vi "Init Tx Packet Size.vi"(8 "error in (no error)":errorcluster, 11 "Tx Loop Data":T1) -> (0 "error out":errorcluster, 3 "Tx Loop Data out":T1)   [LabVIEW 2016, in "UDP-Custom-Device Engine.lvlib"]
uses:
  UDP-Custom-Device Engine.lvlib
  Tx Loop Data.ctl
  <vilib>/NI Veristand/VeriStand Data/Byte Buffer/Byte Buffer.lvclass
  <vilib>/NI/NIVS Inline Async API/_Data Access Engine/Data Access Engine/Types/Read.DVR.ctl
  <vilib>/NI/NIVS Inline Async API/_Data Access Engine/Access Type Classes/Read/Read.lvclass
  <vilib>/NI Veristand/VeriStand Data/Typedefs/Typedefs.Data Types.ctl
  Data Conversion Config.ctl
  <vilib>/NI Veristand/VeriStand Data/Byte Buffer/Byte Buffer.Mapping.ctl
  Shared/Header Details.ctl
  <vilib>/NI/NIVS Inline Async API/_Data Access Engine/Data Access Engine/Data Access Engine.lvclass
  <vilib>/NI Veristand/VeriStand Data/VeriStand Data.lvlib
  Shared/UDP-Custom-Device Shared.lvlib
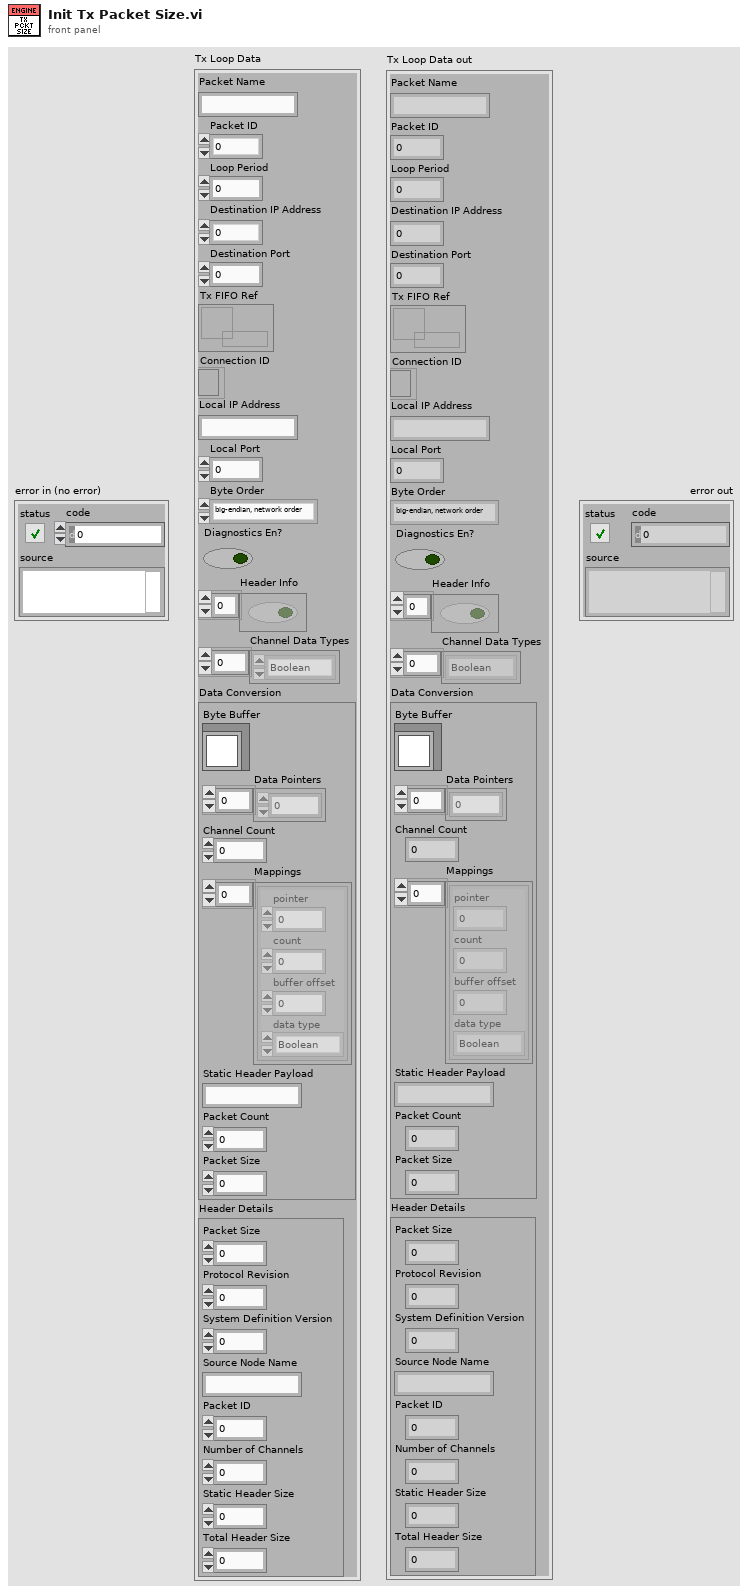
[diagram p1: front panel]
types:
  T1 = typedef "UDP-Custom-Device Engine.lvlib/Tx Loop Data.ctl" = cluster{"Packet Name":string, "Packet ID":i32, "Loop Period":u32, "Destination IP Address":u32, "Destination Port":u16, "Tx FIFO Ref":T2, "Connection ID":refnum<k16>, "Local IP Address":string, "Local Port":i32, "Byte Order":enum16{"big-endian, network order", "native, host order", "little-endian"}, "Diagnostics En?":bool, "Header Info":bool[], "Channel Data Types":T3[], "Data Conversion":T4, "Header Details":T6}
  T2 = typedef "Data Access Engine.lvlib/Data Access Engine.lvclass/Read.DVR.ctl" = refnum<data-value>
  T3 = typedef "VeriStand Data.lvlib/Typedefs.Data Types.ctl" = enum16{"Boolean", "Single", "Double", "I8", "I16", "I32", "I64", "U8", "U16", "U32", "U64"}
  T4 = typedef "UDP-Custom-Device Engine.lvlib/Data Conversion Config.ctl" = cluster{"Byte Buffer":refnum<class "Byte Buffer.lvclass">, "Data Pointers":u64[], "Channel Count":i32, "Mappings":T5[], "Static Header Payload":string, "Packet Count":dbl, "Packet Size":i32}
  T5 = typedef "VeriStand Data.lvlib/Byte Buffer.lvclass/Byte Buffer.Mapping.ctl" = cluster{"pointer":u64, "count":i64, "buffer offset":u64, "data type":T3}
  T6 = typedef "UDP-Custom-Device Shared.lvlib/Header Details.ctl" = cluster{"Packet Size":u16, "Protocol Revision":u8, "System Definition Version":u64, "Source Node Name":string, "Packet ID":u32, "Number of Channels":u32, "Static Header Size":u16, "Total Header Size":u16}
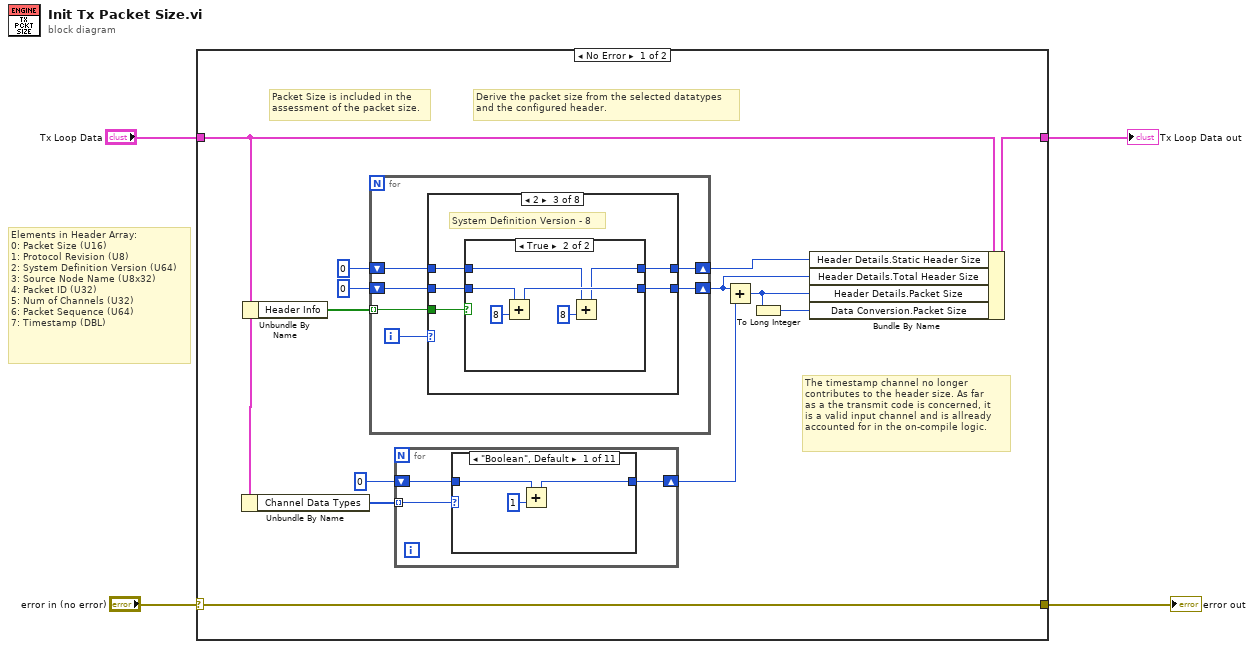
[diagram p0: block diagram]
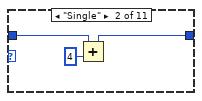
[diagram p2: hidden frame]
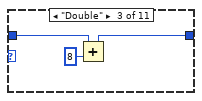
[diagram p3: hidden frame]
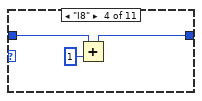
[diagram p4: hidden frame]
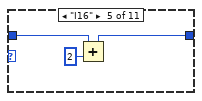
[diagram p5: hidden frame]
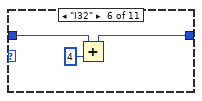
[diagram p6: hidden frame]
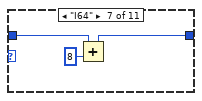
[diagram p7: hidden frame]
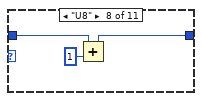
[diagram p8: hidden frame]
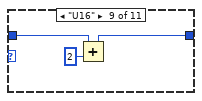
[diagram p9: hidden frame]
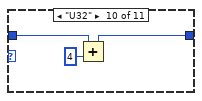
[diagram p10: hidden frame]
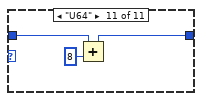
[diagram p11: hidden frame]
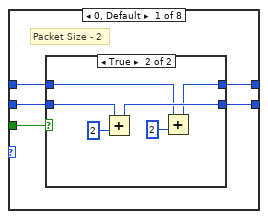
[diagram p12: hidden frame]
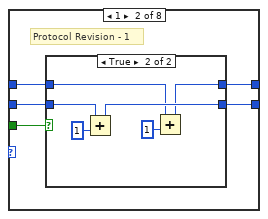
[diagram p14: hidden frame]
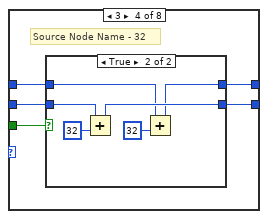
[diagram p17: hidden frame]
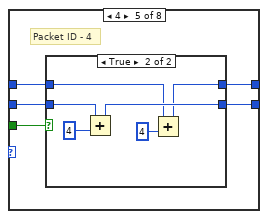
[diagram p19: hidden frame]
diagram:
  # "Elements in Header Array:\n0: Packet Size (U16)\n1: Protocol Revision (U8)\n2: System Definition Version (U64)\n3: Source Node Name (U8x32)\n4: Packet ID (U32)\n5: Num of Channels (U32)\n6: Packet Sequence (U64)\n7: Timestamp (DBL)"
  n1 = case shown="No Error" "error in (no error)" {
    selector: "error in (no error)" -> [w17 w161]
    tunnel: [w17 w161] -> w3
    tunnel: [w16 w160] -> w2
    tunnel: "Tx Loop Data" -> [w14 w160]
    frame No Error {
      # "The timestamp channel no longer\ncontributes to the header size. As far\nas a the transmit code is concerned, it\nis a valid input channel and is allready\naccounted for in the on-compile logic."
      # "Packet Size is included in the\nassessment of the packet size."
      # "Derive the packet size from the selected datatypes\nand the configured header."
      n2 = Unbundle By Name(w14) -> ("Channel Data Types"=w13:T3[])
      n3 = Unbundle By Name(w14) -> ("Header Info"=w15:bool[])
      n4 = for {
        tunnel: w15 -> [w59] mode=indexing
        shift-right: [w56] -> w10
        shift-left: u16 0 -> [w57]
        shift-right: [w54] -> w8
        shift-left: u16 0 -> [w55]
        i -> [w58]
        n5 = case shown="2" w58 {
          tunnel: w59 -> [w64 w77 w90 w103 w116 w129 w142 w153]
          tunnel: w57 -> [w63 w76 w89 w102 w115 w128 w141 w152]
          tunnel: [w62 w75 w88 w101 w114 w127 w140 w151] -> w56
          tunnel: w55 -> [w61 w74 w87 w100 w113 w126 w139 w150]
          tunnel: [w60 w73 w86 w99 w112 w125 w138 w149] -> w54
          frame 0, Default {
            # "Packet Size - 2"
            n6 = case shown="True" w64 {
              tunnel: w63 -> [w66 w72]
              tunnel: [w66 w70] -> w62
              tunnel: w61 -> [w65 w68]
              tunnel: [w65 w67] -> w60
              frame False {
              }
              frame True {
                n7 = Add(x=w72, y=u16 2) -> (x+y=w70:u16)
                n8 = Add(x=w68, y=u16 2) -> (x+y=w67:u16)
              }
            }
          }
          frame 1 {
            # "Protocol Revision - 1"
            n9 = case shown="True" w77 {
              tunnel: w76 -> [w79 w85]
              tunnel: [w79 w83] -> w75
              tunnel: w74 -> [w78 w81]
              tunnel: [w78 w80] -> w73
              frame False {
              }
              frame True {
                n10 = Add(x=w85, y=u16 1) -> (x+y=w83:u16)
                n11 = Add(x=w81, y=u16 1) -> (x+y=w80:u16)
              }
            }
          }
          frame 2 {
            # "System Definition Version - 8"
            n12 = case shown="True" w90 {
              tunnel: w89 -> [w92 w98]
              tunnel: [w92 w96] -> w88
              tunnel: w87 -> [w91 w94]
              tunnel: [w91 w93] -> w86
              frame False {
              }
              frame True {
                n13 = Add(x=w98, y=u16 8) -> (x+y=w96:u16)
                n14 = Add(x=w94, y=u16 8) -> (x+y=w93:u16)
              }
            }
          }
          frame 3 {
            # "Source Node Name - 32"
            n15 = case shown="True" w103 {
              tunnel: w102 -> [w105 w111]
              tunnel: [w105 w109] -> w101
              tunnel: w100 -> [w104 w107]
              tunnel: [w104 w106] -> w99
              frame False {
              }
              frame True {
                n16 = Add(x=w111, y=u16 32) -> (x+y=w109:u16)
                n17 = Add(x=w107, y=u16 32) -> (x+y=w106:u16)
              }
            }
          }
          frame 4 {
            # "Packet ID - 4"
            n18 = case shown="True" w116 {
              tunnel: w115 -> [w118 w124]
              tunnel: [w118 w122] -> w114
              tunnel: w113 -> [w117 w120]
              tunnel: [w117 w119] -> w112
              frame False {
              }
              frame True {
                n19 = Add(x=w124, y=u16 4) -> (x+y=w122:u16)
                n20 = Add(x=w120, y=u16 4) -> (x+y=w119:u16)
              }
            }
          }
          frame 5 {
            # "Num of Channels - 4"
            n21 = case shown="True" w129 {
              tunnel: w128 -> [w131 w137]
              tunnel: [w131 w135] -> w127
              tunnel: w126 -> [w130 w133]
              tunnel: [w130 w132] -> w125
              frame False {
              }
              frame True {
                n22 = Add(x=w137, y=u16 4) -> (x+y=w135:u16)
                n23 = Add(x=w133, y=u16 4) -> (x+y=w132:u16)
              }
            }
          }
          frame 6 {
            # "Packet Sequence - 8"
            n24 = case shown="True" w142 {
              tunnel: w141 -> [w144 w148]
              tunnel: [w144 w146] -> w140
              tunnel: w139 -> [w143 w145]
              tunnel: [w143 w145] -> w138
              frame False {
              }
              frame True {
                n25 = Add(x=w148, y=u16 8) -> (x+y=w146:u16)
              }
            }
          }
          frame 7 {
            # "Timestamp - 8"
            n26 = case shown="True" w153 {
              tunnel: w152 -> [w155 w159]
              tunnel: [w155 w157] -> w151
              tunnel: w150 -> [w154 w156]
              tunnel: [w154 w156] -> w149
              frame False {
              }
              frame True {
                n27 = Add(x=w159, y=u16 0) -> (x+y=w157:u16)
              }
            }
          }
        }
      }
      n28 = for {
        tunnel: w13 -> [w20] mode=indexing
        shift-right: [w18] -> w6
        shift-left: u16 0 -> [w19]
        n29 = case shown="\"Boolean\", Default" w20 {
          tunnel: w19 -> [w23 w26 w29 w32 w35 w38 w41 w44 w47 w50 w53]
          tunnel: [w21 w24 w27 w30 w33 w36 w39 w42 w45 w48 w51] -> w18
          frame "Boolean", Default {
            n30 = Add(x=w23, y=u16 1) -> (x+y=w21:u16)
          }
          frame "Single" {
            n31 = Add(x=w26, y=u16 4) -> (x+y=w24:u16)
          }
          frame "Double" {
            n32 = Add(x=w29, y=u16 8) -> (x+y=w27:u16)
          }
          frame "I8" {
            n33 = Add(x=w32, y=u16 1) -> (x+y=w30:u16)
          }
          frame "I16" {
            n34 = Add(x=w35, y=u16 2) -> (x+y=w33:u16)
          }
          frame "I32" {
            n35 = Add(x=w38, y=u16 4) -> (x+y=w36:u16)
          }
          frame "I64" {
            n36 = Add(x=w41, y=u16 8) -> (x+y=w39:u16)
          }
          frame "U8" {
            n37 = Add(x=w44, y=u16 1) -> (x+y=w42:u16)
          }
          frame "U16" {
            n38 = Add(x=w47, y=u16 2) -> (x+y=w45:u16)
          }
          frame "U32" {
            n39 = Add(x=w50, y=u16 4) -> (x+y=w48:u16)
          }
          frame "U64" {
            n40 = Add(x=w53, y=u16 8) -> (x+y=w51:u16)
          }
        }
      }
      n41 = Add(x=w10, y=w6) -> (x+y=w5:u16)
      n42 = To Long Integer(number=w5) -> (32bit integer=w7:i32)
      n43 = Bundle By Name(cluster=w14, "Header Details.Static Header Size"=w8, "Header Details.Total Header Size"=w10, "Header Details.Packet Size"=w5, "Data Conversion.Packet Size"=w7) -> (w16:T1)
    }
    frame Error {
    }
  }
  "error out" <- w3
  "Tx Loop Data out" <- w2
